vi "OpenCode.vi"(3 "Code name":string) -> ()   [LabVIEW 2012]
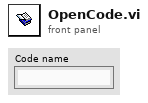
[diagram p1: front panel]
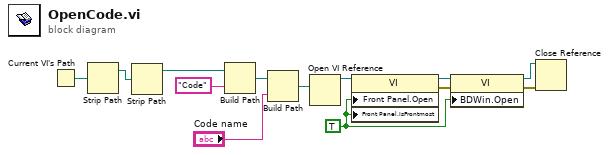
[diagram p0: block diagram]
diagram:
  w10 = TRUE ("Front Panel Window:Open")
  n1 = Current VI's Path() -> (path=w3:path)
  n2 = Strip Path(path=w3) -> (stripped path=w2:path)  [unwired: 1 out]
  n3 = Strip Path(path=w2) -> (stripped path=w1:path)  [unwired: 1 out]
  n4 = Build Path(base path=w1, name or relative path="Code") -> (appended path=w5:path)
  n5 = Build Path(base path=w5, name or relative path="Code name") -> (appended path=w7:path)
  n6 = Open VI Reference(vi path=w7) -> (vi reference=w11:refnum<vi>)  [unwired: 5 in, 1 out]
  n7 = property class="VI"(reference=w11, "Front Panel.Open"=w10, "Front Panel.IsFrontmost"=w10) -> (reference out=w8:refnum<vi>, error out=w9:errorcluster)  [unwired: 1 in]
  n8 = property class="VI"(reference=w8, error in=w9, "BDWin.Open"=w10) -> (reference out=w13:refnum<vi>, error out=w12:errorcluster)
  n9 = Close Reference(reference=w13, error in (no error)=w12) -> ()  [unwired: 1 out]
